vi "TPNT_ReadDataFromFile.vi"(8 "error in (no error)":errorcluster, 11 "TPs directory":path) -> (0 "error out":errorcluster)   [LabVIEW 2016]
uses:
  TPNT_DeviceTPs.ctl
  TPNT_TP.ctl
  TPNT_Limits.ctl
  TPNT_Samples.ctl
  TPNT_Log.ctl
  <vilib>/Utility/config.llb/Read Key (String).vi
  <vilib>/Utility/config.llb/NI_LVConfig.lvlib
panel:
  in  "TPNT_TP":T1={"name"="", "type"="", "algor"=[], "update_rate"=0.0, "Limits"={"Alarm Type"="", "Lower "=0.0, "Upper"=0.0, "Nominal"=0.0, "outrange"=FALSE, "Check"=TRUE, "latch"=FALSE, "level"=""}, "Samples"={"samples"=0, "counter"=0, "Values"=[], "Current Value"="", "filter"="", "precision"=2}, "next_update"=0, "Status"="", "monitor"=TRUE, "error"=FALSE, "Log"={"log"=FALSE, "file"=path "", "type"="", "format"="", "updaterate"=0.0, "nex_update"=0, "mode"=""}, "permissions"="", "ID"=""} {"Log"."updaterate" format="%.2f"; "Samples"."Values" format="%.2f"; "Samples"."samples" min=1 step=1; "Limits"."Nominal" format="%.2f"; "Limits"."Upper" format="%.2f"; "Limits"."Lower" format="%.2f"; "update_rate" format="%.2f"}
  in  "TPNT_DeviceTPs":T5={"device"="", "devupdate"=0.0, "next_update"=0, "devinterface"="", "TPs"=[], "Alarms"=TRUE, "monitor"=TRUE, "log sep"=""} {"TPs"."Log"."updaterate" format="%.2f"; "TPs"."Samples"."Values" format="%.2f"; "TPs"."Samples"."samples" min=1 step=1; "TPs"."Limits"."Nominal" format="%.2f"; "TPs"."Limits"."Upper" format="%.2f"; "TPs"."Limits"."Lower" format="%.2f"; "TPs"."update_rate" format="%.2f"; "devupdate" format="%.2f"}
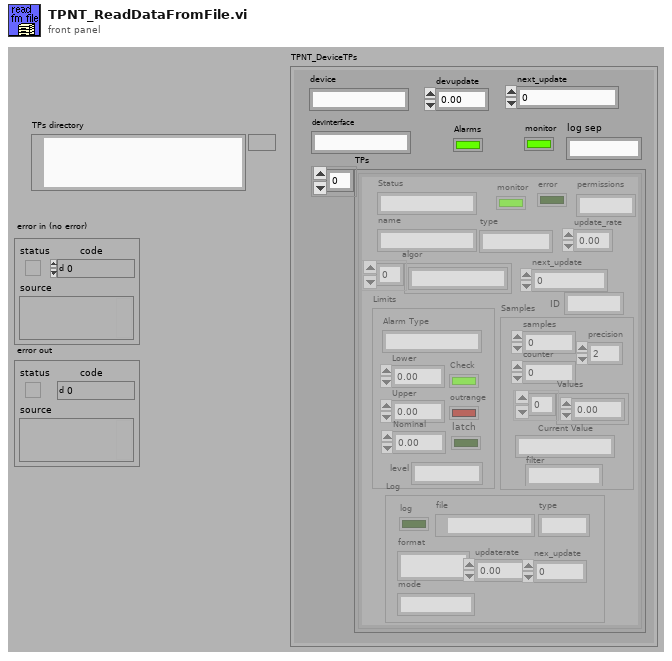
[diagram p1: front panel]
types:
  T1 = typedef "TPNT_TP.ctl" = cluster{"name":string, "type":string, "algor":string[], "update_rate":sgl, "Limits":T2, "Samples":T3, "next_update":u32, "Status":string, "monitor":bool, "error":bool, "Log":T4, "permissions":string, "ID":string}
  T2 = typedef "TPNT_Limits.ctl" = cluster{"Alarm Type":string, "Lower ":dbl, "Upper":dbl, "Nominal":dbl, "outrange":bool, "Check":bool, "latch":bool, "level":string}
  T3 = typedef "TPNT_Samples.ctl" = cluster{"samples":i32, "counter":i32, "Values":dbl[], "Current Value":string, "filter":string, "precision":u8}
  T4 = typedef "TPNT_Log.ctl" = cluster{"log":bool, "file":path, "type":string, "format":string, "updaterate":dbl, "nex_update":u32, "mode":string}
  T5 = typedef "TPNT_DeviceTPs.ctl" = cluster{"device":string, "devupdate":dbl, "next_update":u32, "devinterface":string, "TPs":T1[], "Alarms":bool, "monitor":bool, "log sep":string}
  T6 = typedef "NI_LVConfig.lvlib/Config Data RefNum.ctl" = refnum<k1>
  T7 = typedef "TPNT_Refnum.ctl" = refnum<vi>
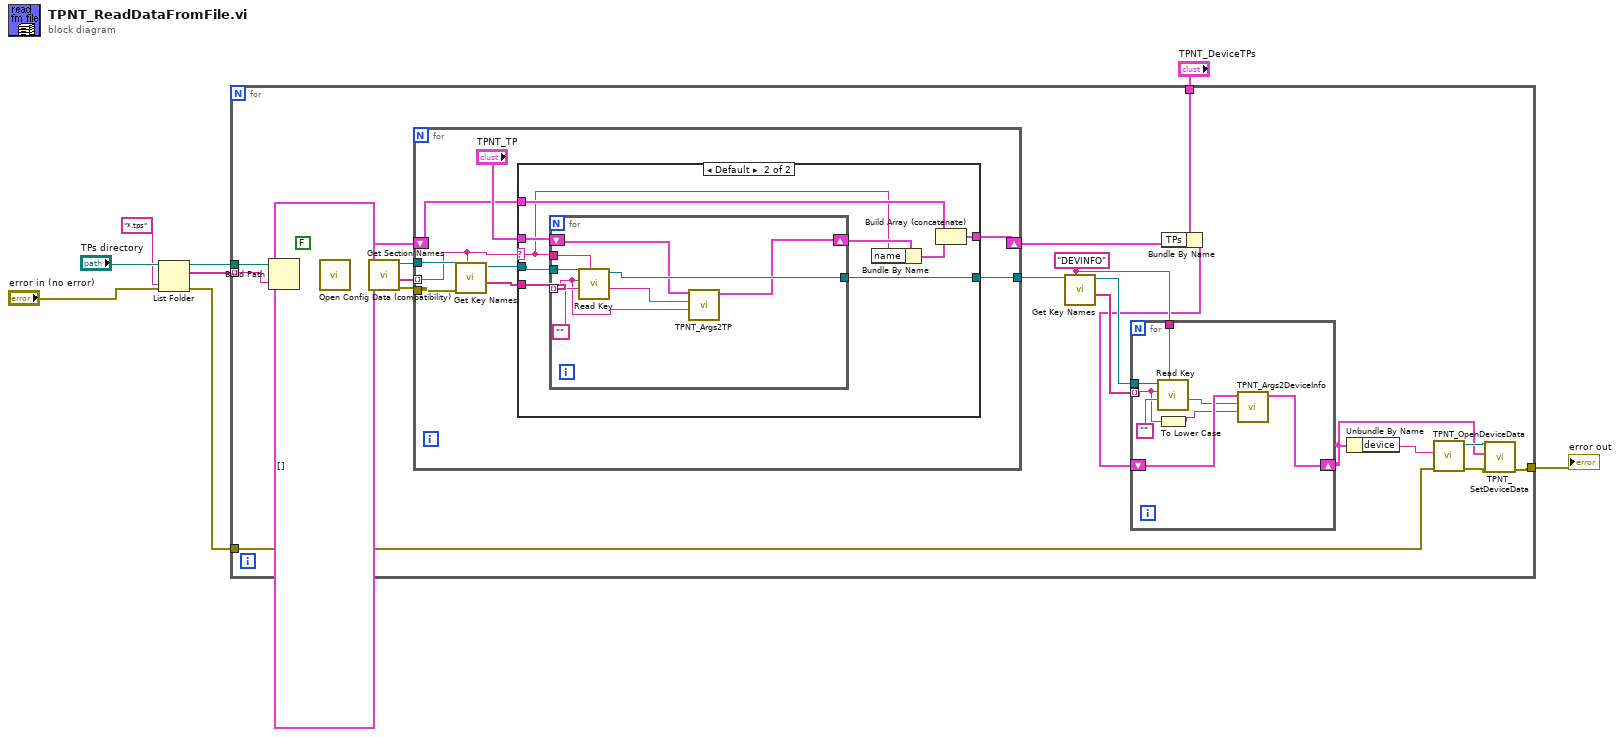
[diagram p0: block diagram]
diagram:
  n1 = List Folder(path="TPs directory", pattern="*.tps", error in="error in (no error)") -> (path out=w5:path, filenames=w6:string[], error out=w1:errorcluster)  [unwired: 2 out]
  n2 = for {
    tunnel: w6 -> [w30] mode=indexing
    tunnel: w5 -> [w31]
    tunnel: "TPNT_DeviceTPs" -> [w16]
    tunnel: [w10] -> w2
    tunnel: w1 -> [w13]
    w18 = "DEVINFO" ("section")
    n3 = Build Path(base path=w31, name or relative path=w30) -> (appended path=w29:path)
    n4 = call <vilib>:"Open Config Data (compatibility).vi"("create file if necessary (T)"=FALSE ("create file if necessary? (T)"), "configuration file path"=w29) -> ("error out"=w26:errorcluster, "refnum"=w27:T6)  [unwired: 7 in, 1 out]
    n5 = call <vilib>:"Get Section Names.vi"("error in (no error)"=w26, "refnum"=w27) -> ("error out"=w23:errorcluster, "section names"=w24:string[], "refnum out"=w25:T6)  [unwired: 7 out]
    n6 = for {
      tunnel: w25 -> [w48]
      tunnel: w23 -> [w47]
      tunnel: w24 -> [w40] mode=indexing
      tunnel: [w43] -> w22
      shift-right: [w41] -> w17
      shift-left: T1[] [] -> [w42]
      n7 = call <vilib>:"Get Key Names.vi"("section"=w40, "error in (no error)"=w47, "refnum"=w48) -> ("key names"=w46:string[], "refnum out"=w45:T6)  [unwired: 7 out]
      n8 = case shown="Default" w40 {
        selector: w40 -> [_ w51]
        tunnel: w46 -> [_ w59]
        tunnel: w45 -> [w49 w58]
        tunnel: "TPNT_TP" -> [_ w57]
        tunnel: [w49 w55] -> w43
        tunnel: w42 -> [w50 w53]
        tunnel: [w50 w52] -> w41
        frame "DEVINFO", "INFO" {
        }
        frame Default {
          n9 = for {
            tunnel: w59 -> [w63] mode=indexing
            tunnel: w51 -> [w65]
            tunnel: w58 -> [w67]
            shift-right: [w60] -> w56
            shift-left: w57 -> [w61]
            tunnel: [w64] -> w55
            n10 = call-poly <vilib>:"Read Key.vi"("section"=w65, "default value"="", "key"=w63, "refnum"=w67) -> ("value"=w62:string, "refnum out"=w64:T6)  [unwired: 2 in, 4 out]
            n11 = call "TPNT_Args2TP.vi"("key"=w63, "value"=w62, "TP_IN"=w61) -> ("TP_OUT"=w60:T1)  [unwired: 8 out]
          }
          n12 = Bundle By Name(cluster=w56, "name"=w51) -> (w54:T1)
          n13 = Build Array (concatenate)(w53, w54) -> (w52:T1[])
        }
      }
    }
    n14 = call <vilib>:"Get Key Names.vi"("section"=w18, "refnum"=w22) -> ("key names"=w20:string[], "refnum out"=w19:T6)  [unwired: 1 in, 7 out]
    n15 = Bundle By Name(cluster=w16, "TPs"=w17) -> (w15:T5)
    n16 = for {
      tunnel: w20 -> [w36] mode=indexing
      tunnel: w19 -> [w39]
      tunnel: w18 -> [w38]
      shift-right: [w34] -> w9
      shift-left: w15 -> [w35]
      n17 = call-poly <vilib>:"Read Key.vi"("section"=w38, "default value"="", "key"=w36, "refnum"=w39) -> ("value"=w33:string)  [unwired: 2 in, 5 out]
      n18 = To Lower Case(string=w36) -> (all lower case string=w32:string)
      n19 = call "TPNT_Args2DeviceInfo.vi"("key"=w32, "value"=w33, "Device IN"=w35) -> ("Device OUT"=w34:T5)  [unwired: 8 out]
    }
    n20 = Unbundle By Name(w9) -> ("device"=w14:string)
    n21 = call "TPNT_OpenDeviceData.vi"("error in (no error)"=w13, "Name"=w14) -> ("error out"=w12:errorcluster, "Data Refnum out"=w11:T7)  [unwired: 8 out]
    n22 = call "TPNT_SetDeviceData.vi"("error in (no error)"=w12, "Object Data In"=w9, "Object Refnum In"=w11) -> ("error out"=w10:errorcluster)  [unwired: 8 out]
  }
  "error out" <- w2
